vi "API - Read 1 Analog Input Sample on Demand.vi"(8 "error in":errorcluster, 10 "Analog Input Channel Number":i32, 11 "TCP Network Connection in":refnum<k5>) -> (0 "error out":errorcluster, 2 "Data Out":dbl, 3 "TCP Network Connection out":refnum<k5>)   [LabVIEW 2020]
doc: "Read a single ADC measurement from the DAQ.\n-Enable channel\n-Start streaming of data\n-Download 1 datapoint\n-Stop streaming of data"
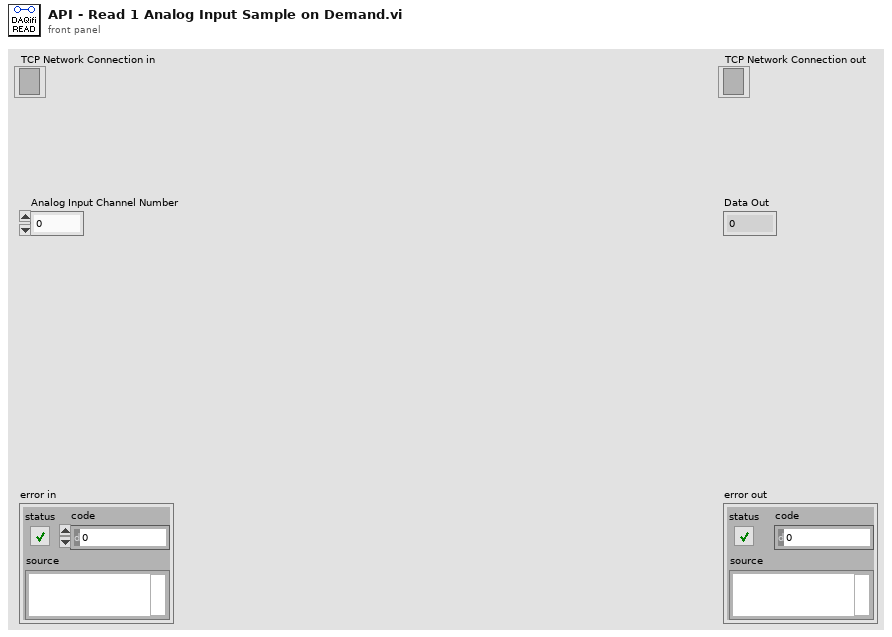
[diagram p1: front panel]
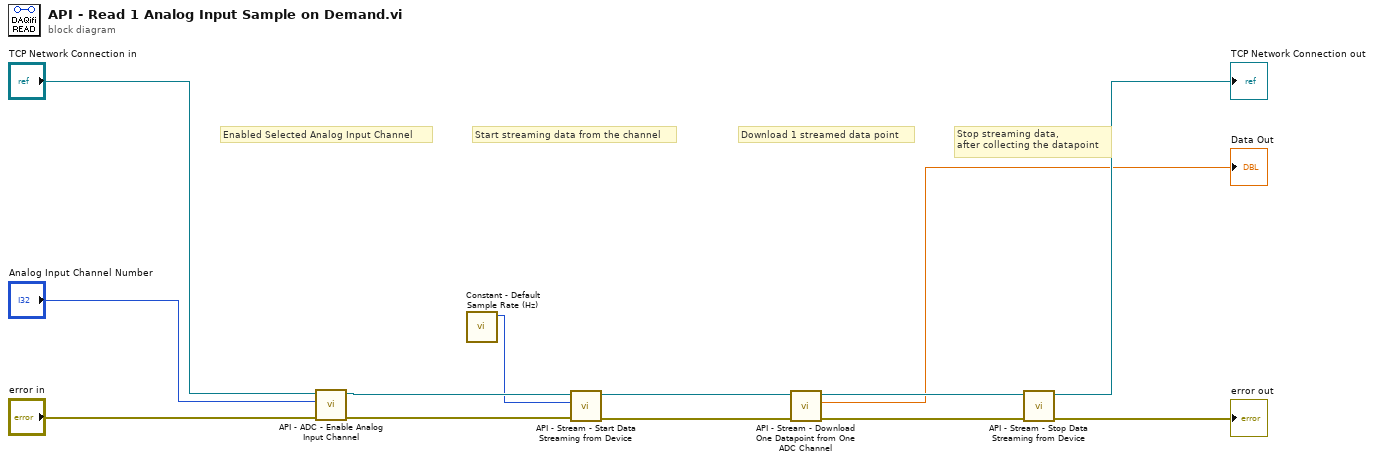
[diagram p0: block diagram]
diagram:
  # "Download 1 streamed data point"
  # "Enabled Selected Analog Input Channel"
  # "Stop streaming data,\nafter collecting the datapoint"
  # "Start streaming data from the channel"
  n1 = call "API - ADC - Enable Analog Input Channel.vi"("error in (no error)"="error in", "Analog Input Channel Number"="Analog Input Channel Number", "TCP Network Connection in"="TCP Network Connection in") -> ("error out"=w2:errorcluster, "TCP Network Connection out"=w3:refnum<k5>)  [unwired: 7 in]
  n2 = call "Constant - Default Sample Rate (Hz).vi"() -> ("Streaming Rate (Hz)"=w1:i32)  [unwired: 11 in]
  n3 = call "API - Stream - Start Data Streaming from Device.vi"("error in (no error)"=w2, "Streaming Rate (Hz)"=w1, "TCP Network Connection in"=w3) -> ("error out"=w8:errorcluster, "TCP Network Connection out"=w9:refnum<k5>)  [unwired: 7 in]
  n4 = call "API - Stream - Download One Datapoint from One ADC Channel.vi"("error in"=w8, "TCP Network Connection in"=w9) -> ("error out"=w12:errorcluster, "Analog Voltage (V)"=→"Data Out":dbl, "TCP Network Connection out"=w13:refnum<k5>)  [unwired: 7 in]
  n5 = call "API - Stream - Stop Data Streaming from Device.vi"("error in (no error)"=w12, "TCP Network Connection in"=w13) -> ("error out"=→"error out":errorcluster, "TCP Network Connection out"=→"TCP Network Connection out":refnum<k5>)  [unwired: 8 in]
